vi "unpackMeterPara.vi"(6 "长度":i32, 7 "数据":u8[](array[numeric]) format="%.0x") -> (2 "输入通道":u8, 3 "电能表参数":T1)   [LabVIEW 2014]
panel:
  out "告警信息":string
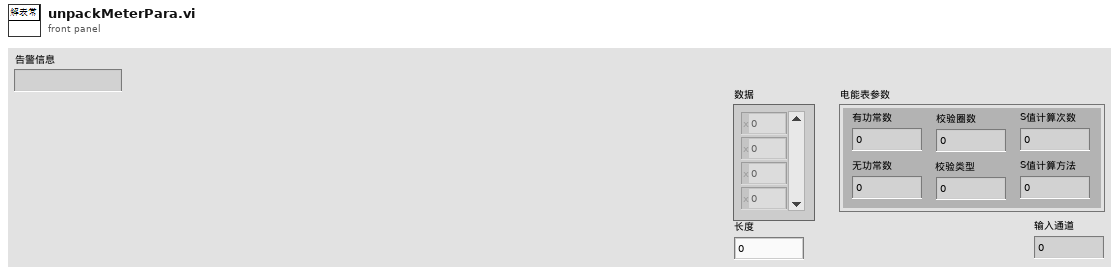
[diagram p1: front panel]
types:
  T1 = cluster{"有功常数":i32, "无功常数":i32, "校验圈数":i32, "校验类型":i32, "S值计算次数":i32, "S值计算方法":i32}
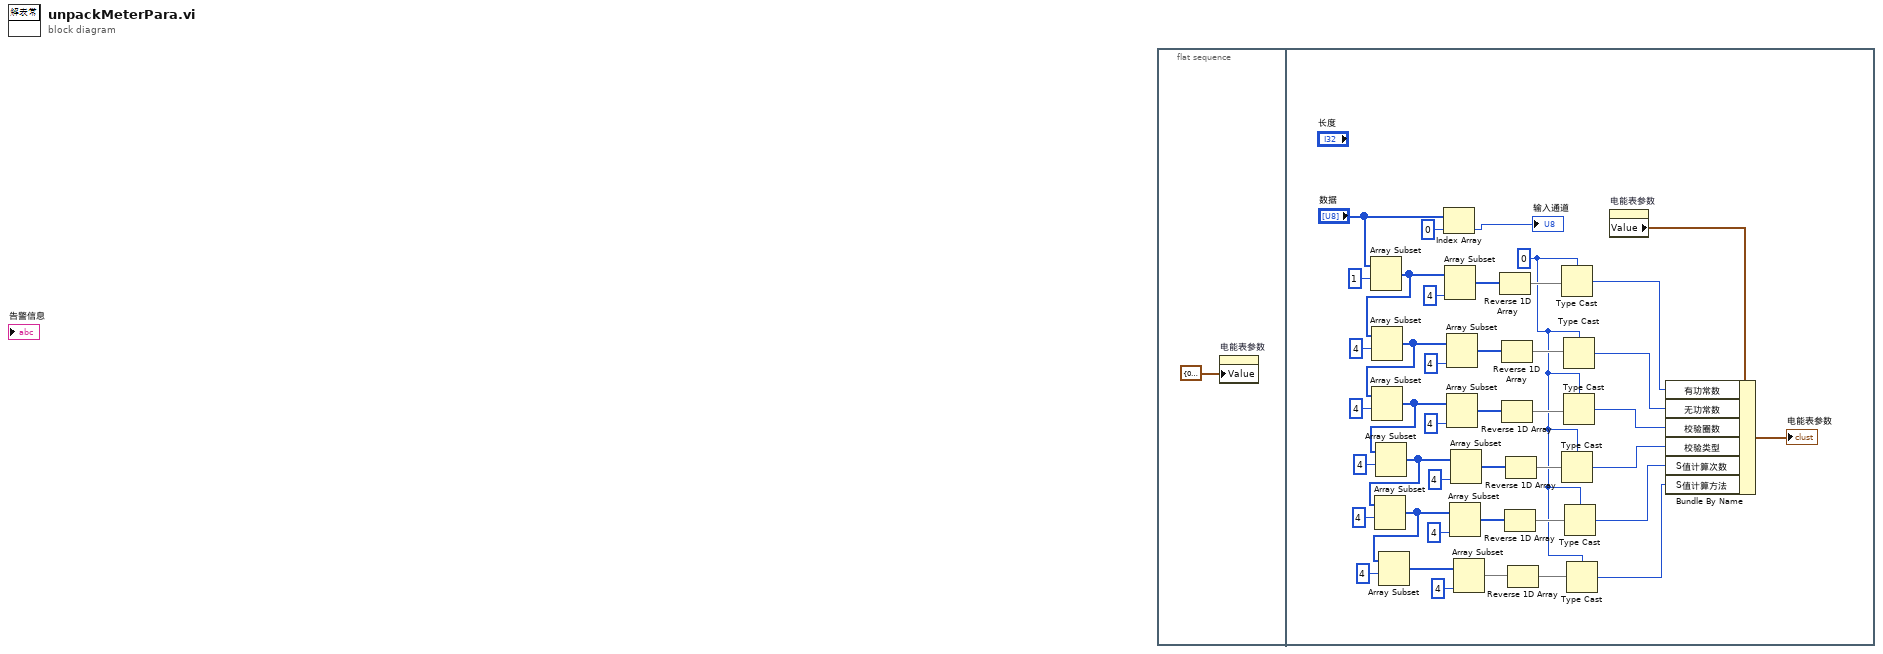
[diagram p0: block diagram]
diagram:
  n1 = flat-sequence {
    frame #0 {
      n2 = property on="电能表参数" class="Clust (严格)"("Value"=T1 {"有功常数"=0, "无功常数"=0, "校验圈数"=0, "校验类型"=0, "S值计算次数"=0, "S值计算方法"=0} ("电能表参数")) -> ()  [unwired: 2 in, 2 out]
    }
    frame #1 {
      w11 = 0
      n3 = Array Subset(array="数据", index=1 ("索引")) -> (w35:u8[])  [unwired: 1 in]
      n4 = Array Subset(array=w35, index=4 ("索引")) -> (w31:u8[])  [unwired: 1 in]
      n5 = Array Subset(array=w31, index=4 ("索引")) -> (w27:u8[])  [unwired: 1 in]
      n6 = Array Subset(array=w27, index=4 ("索引")) -> (w18:u8[])  [unwired: 1 in]
      n7 = Array Subset(array=w18, index=4 ("索引")) -> (w26:u8[])  [unwired: 1 in]
      n8 = Array Subset(array=w26, index=4 ("索引")) -> (w25:u8[])  [unwired: 1 in]
      n9 = Index Array(array="数据", index=0 ("索引")) -> (element=→"输入通道":u8)
      n10 = Array Subset(array=w35, length=4 ("长度")) -> (w41:u8[])  [unwired: 1 in]
      n11 = Array Subset(array=w31, length=4 ("长度")) -> (w40:u8[])  [unwired: 1 in]
      n12 = Array Subset(array=w27, length=4 ("长度")) -> (w32:u8[])  [unwired: 1 in]
      n13 = Array Subset(array=w26, length=4 ("长度")) -> (w21:u8[])  [unwired: 1 in]
      n14 = Array Subset(array=w18, length=4 ("长度")) -> (w30:u8[])  [unwired: 1 in]
      n15 = Array Subset(array=w25, length=4 ("长度")) -> (w22:u8[])  [unwired: 1 in]
      n16 = Reverse 1D Array(array=w41) -> (reversed array=w17:u8[])
      n17 = Reverse 1D Array(array=w40) -> (reversed array=w16:u8[])
      n18 = Reverse 1D Array(array=w32) -> (reversed array=w15:u8[])
      n19 = Reverse 1D Array(array=w21) -> (reversed array=w13:u8[])
      n20 = Reverse 1D Array(array=w30) -> (reversed array=w14:u8[])
      n21 = Reverse 1D Array(array=w22) -> (reversed array=w12:u8[])
      n22 = Type Cast(type=w11, x=w17) -> (*(type *) &x=w9:i32)
      n23 = Type Cast(type=w11, x=w14) -> (*(type *) &x=w6:i32)
      n24 = Type Cast(type=w11, x=w16) -> (*(type *) &x=w8:i32)
      n25 = Type Cast(type=w11, x=w15) -> (*(type *) &x=w7:i32)
      n26 = Type Cast(type=w11, x=w13) -> (*(type *) &x=w5:i32)
      n27 = Type Cast(type=w11, x=w12) -> (*(type *) &x=w4:i32)
      n28 = property on="电能表参数" class="Clust (严格)"() -> ("Value"=w10:T1)  [unwired: 2 in, 2 out]
      n29 = Bundle By Name(cluster=w10, "有功常数"=w9, "无功常数"=w8, "校验圈数"=w7, "校验类型"=w6, "S值计算次数"=w5, "S值计算方法"=w4) -> (→"电能表参数":T1)
    }
  }
